vi "Drive_Loop_Command.vi"   [LabVIEW 2016]
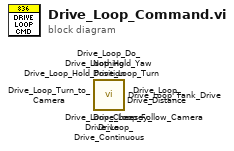
[diagram p0: block diagram]
diagram:
  n1 = call <userlib>:"Drive_Loop_Cheesey_Drive.vi"() -> ()  [unwired: 12 in]
  n2 = call <userlib>:"Drive_Loop_Turn.vi"() -> ()  [unwired: 12 in]
  n3 = call <userlib>:"Drive_Loop_Turn_to_Camera.vi"() -> ()  [unwired: 12 in]
  n4 = call <userlib>:"Drive_Loop_Tank_Drive.vi"() -> ()  [unwired: 12 in]
  n5 = call <userlib>:"Drive_Loop_Hold_Yaw.vi"() -> ()  [unwired: 12 in]
  n6 = call <userlib>:"Drive_Loop_Hold_Position.vi"() -> ()  [unwired: 12 in]
  n7 = call <userlib>:"Drive_Loop_Follow_Camera.vi"() -> ()  [unwired: 12 in]
  n8 = call <userlib>:"Drive_Loop_Drive_Distance.vi"() -> ()  [unwired: 12 in]
  n9 = call <userlib>:"Drive_Loop_Drive_Continuous.vi"() -> ()  [unwired: 12 in]
  n10 = call <userlib>:"Drive_Loop_Do_Nothing.vi"() -> ()  [unwired: 12 in]
